vi "Read ID.vi"(8 "error in (no error)":errorcluster, 11 "Impot in":refnum<class "Impot.lvclass">) -> (0 "error out":errorcluster, 2 "ID 2":T1, 3 "Impot out":refnum<class "Impot.lvclass">)   [LabVIEW 2023, in "Impot.lvclass"]
uses:
  Impot.lvclass
  Controller/Ctrl_ID.ctl
  Impot.lvclass/Impot.ctl
  ID/ID.lvclass
panel:
  out "ID":T2
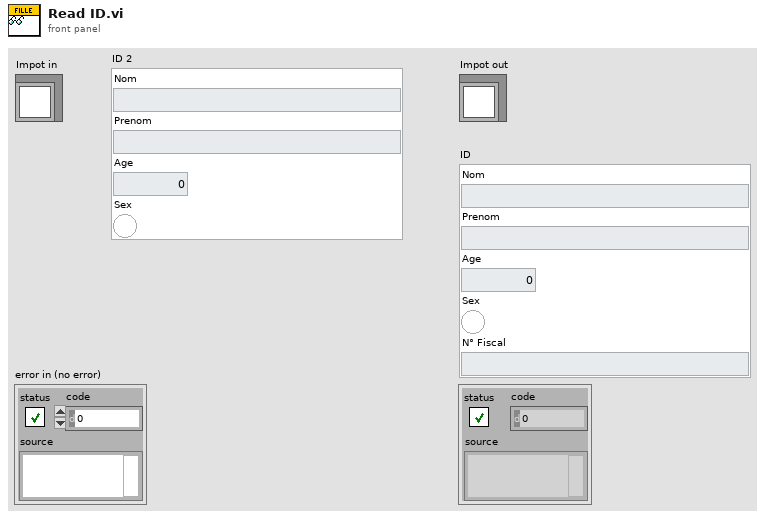
[diagram p1: front panel]
types:
  T1 = typedef "Ctrl_ID.ctl" = cluster{"Nom":string, "Prenom":string, "Age":u8, "Sex":bool}
  T2 = cluster{"Nom":string, "Prenom":string, "Age":u8, "Sex":bool, "N° Fiscal":string}
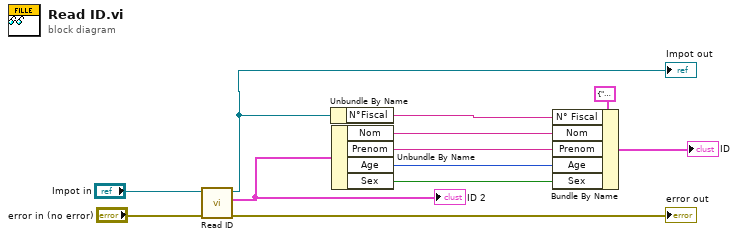
[diagram p0: block diagram]
diagram:
  n1 = call-parent "Read ID.vi"("error in (no error)"="error in (no error)", "ID in"="Impot in") -> ("error out"=→"error out":errorcluster, "ID"=w1:T1, "ID out"=w9:refnum<class "Impot.lvclass">)  [unwired: 7 in]
  "Impot out" <- w9
  "ID 2" <- w1
  n2 = Unbundle By Name(w9) -> ("N°Fiscal"=w7:string)
  n3 = Unbundle By Name(w1) -> ("Nom"=w6:string, "Prenom"=w5:string, "Age"=w4:u8, "Sex"=w3:bool)
  n4 = Bundle By Name(cluster=T2 {"Nom"="", "Prenom"="", "Age"=0, "Sex"=FALSE, "N° Fiscal"=""} ("ID"), "N° Fiscal"=w7, "Nom"=w6, "Prenom"=w5, "Age"=w4, "Sex"=w3) -> (→"ID":T2)
